vi "Determine Warnings.vi"(8 "entrée d'erreur (pas d'erreur)":errorcluster, 9 "Temp. min.":dbl, 10 "Temp. max.":dbl, 11 "Temp. actuelle":dbl) -> (0 "sortie d'erreur":errorcluster, 1 "Mise en garde ?":bool, 2 "Texte de mise en garde":string)   [LabVIEW 2013]
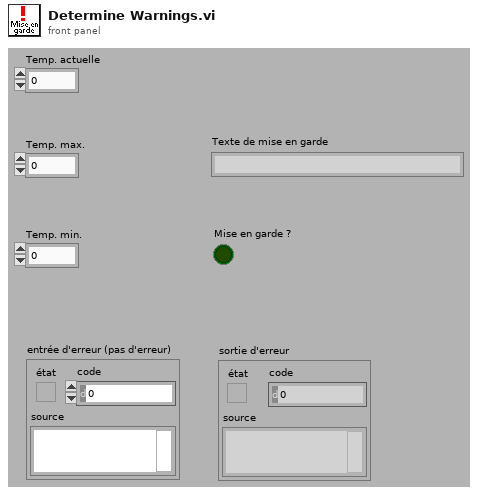
[diagram p1: front panel]
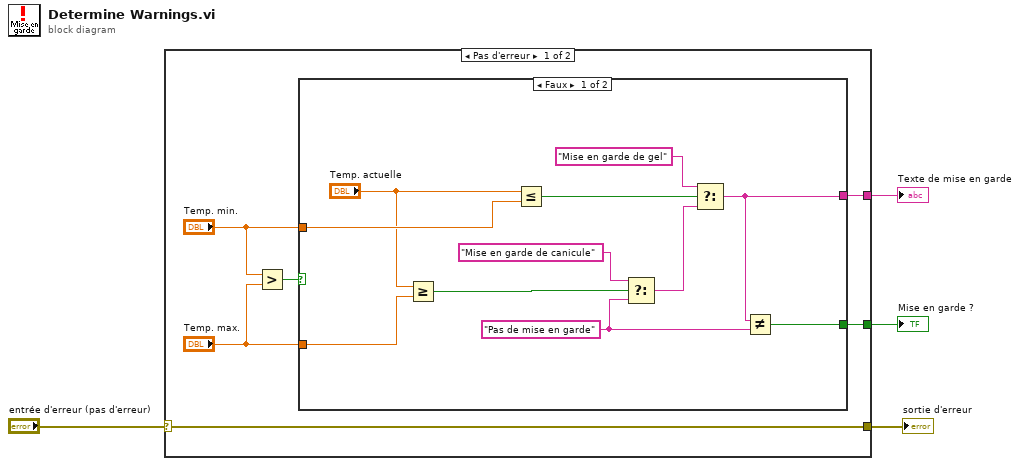
[diagram p0: block diagram]
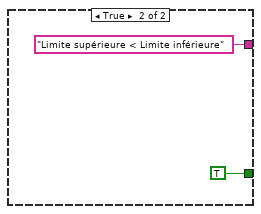
[diagram p2: hidden frame]
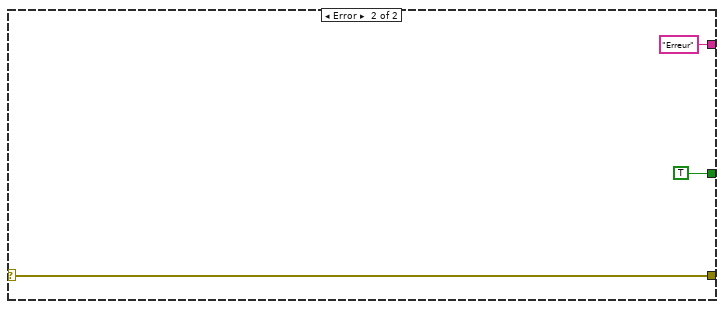
[diagram p3: hidden frame]
diagram:
  n1 = case "Structure Condition" shown="Pas d'erreur" "entrée d'erreur (pas d'erreur)" {
    selector: "entrée d'erreur (pas d'erreur)" -> [w5 w26]
    tunnel: [w10 "Erreur" ("f")] -> w4
    tunnel: [w9 TRUE] -> w3
    tunnel: [w5 w26] -> w1
    frame No Error {
      n2 = Greater? ("Supérieur ?")(x="Temp. min.", y="Temp. max.") -> (0:w8:bool)
      n3 = case "Structure Condition" shown="Faux" w8 {
        tunnel: [w21 "Limite supérieure < Limite inférieure" ("f")] -> w10
        tunnel: [w20 TRUE] -> w9
        tunnel: "Temp. max." -> [w19 _]
        tunnel: "Temp. min." -> [w16 _]
        frame False {
          w11 = "Pas de mise en garde" ("f")
          n4 = Greater Or Equal?(x="Temp. actuelle", y=w19) -> (x >= y?=w18:bool)
          n5 = Less Or Equal?(x="Temp. actuelle", y=w16) -> (x <= y?=w13:bool)
          n6 = Select(t="Mise en garde de canicule", s=w18, f=w11) -> (s? t:f=w12:string)
          n7 = Select(t="Mise en garde de gel", s=w13, f=w12) -> (s? t:f=w21:string)
          n8 = Not Equal?(x=w21, y=w11) -> (x != y?=w20:bool)
        }
        frame True {
        }
      }
    }
    frame Error {
    }
  }
  "Texte de mise en garde" <- w4
  "Mise en garde ?" <- w3
  "sortie d'erreur" <- w1
